vi "Remove.vi"(8 "error in (no error)":errorcluster, 11 "Recipe Step in":refnum<class "Recipe Step.lvclass">) -> (0 "error out":errorcluster, 3 "Recipe Step out":refnum<class "Recipe Step.lvclass">)   [LabVIEW 2018, in "Temp Recipe.lvlib" / "Recipe Step.lvclass"]
uses:
  Recipe Step.lvclass
  C:/dev/source/Libraries/OOPanel/OOPanel/Panel/Panel.lvclass
  Recipe Step.lvclass/Recipe Step.ctl
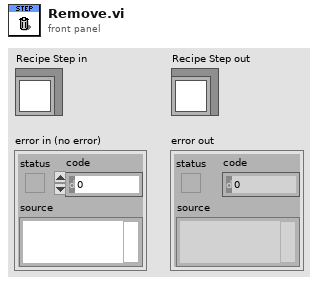
[diagram p1: front panel]
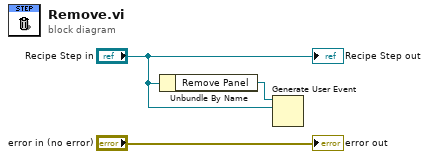
[diagram p0: block diagram]
diagram:
  n1 = Unbundle By Name("Recipe Step in") -> ("Remove Panel"=w2:refnum<user-event>)
  n2 = Generate User Event(user event=w2, event data cluster="Recipe Step in") -> ()  [unwired: 2 in, 2 out]
  "error out" <- "error in (no error)"
  "Recipe Step out" <- "Recipe Step in"
